vi "FTW-Example-EventLogger.vi"() -> ()   [LabVIEW 2015]
uses:
  source/actor/EventLogger/FTW-Logger.lvclass
  source/actor/Ether/FTW-Ether.lvclass
panel:
  in  "FTW Ether Configuration":string="{\n  \"ApplicationName\": \"Logger Example\",\n  \"ApplicationVersion\": \"0.1.0-1\",\n  \"LoggerAddress\": \"inproc://*\",\n  \"LoggerName\": \"LoggerExample\",\n  \"LoggerDirectory\": \"[UserDesktop]\\\\Logs\",\n  \"LoggerDiskThrashDelay\": 200\n}"
  in  "Logger Configuration":string="{\n  \"Identity\": \"EventLog\",\n  \"InboxAddress\": \"inproc://*\",\n  \"LoggerAddress\": \"\",\n  \"DebugEnableInboxLogging\": false,\n  \"DebugEnableJobLogging\": false,\n  \"DebugShowPanel\": false,\n  \"ApplicationName\": \"LoggerExample\",\n  \"LoggerName\": \"SecondLogger\",\n  \"LoggerDirectory\": \"[UserDesktop]\\\\Logs\",\n  \"LoggerDiskThrashDelay\": 200\n}"
  out "error out":errorcluster
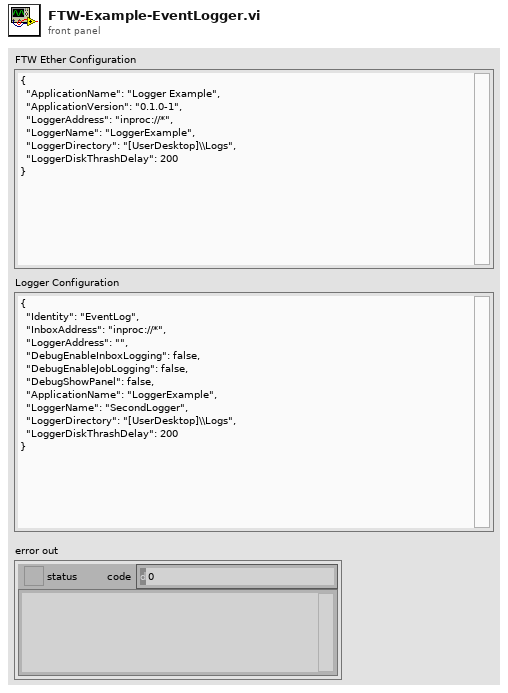
[diagram p1: front panel]
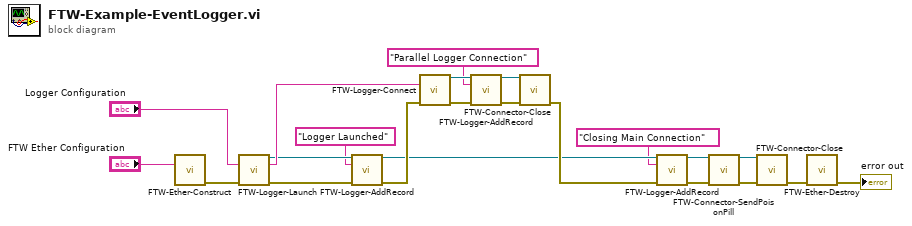
[diagram p0: block diagram]
diagram:
  n1 = call "FTW-Ether-Construct.vi"("FTW Ether Configuration"="FTW Ether Configuration") -> ("error out"=w4:errorcluster)  [unwired: 14 in]
  n2 = call "FTW-Logger-Launch.vi"("FTW Logger Configuration"="Logger Configuration", "error in"=w4) -> ("FTW Logger Connector"=w16:refnum<class "FTW-Logger.lvclass">, "Logger Address"=w18:string, "error out"=w15:errorcluster)  [unwired: 10 in, 1 out]
  n3 = call "FTW-Logger-AddRecord.vi"("FTW Logger Connector"=w16, "Event Type"="Logger Launched", "error in"=w15) -> ("FTW Logger Connector out"=w10:refnum<class "FTW-Logger.lvclass">, "error out"=w14:errorcluster)  [unwired: 10 in, 1 out]
  n4 = call "FTW-Logger-Connect.vi"("Logger Address"=w18, "error in"=w14) -> ("FTW Logger Connector"=w21:refnum<class "FTW-Logger.lvclass">, "error out"=w19:errorcluster)  [unwired: 12 in]
  n5 = call "FTW-Logger-AddRecord.vi"("FTW Logger Connector"=w21, "Event Type"="Parallel Logger Connection", "error in"=w19) -> ("FTW Logger Connector out"=w12:refnum<class "FTW-Logger.lvclass">, "error out"=w11:errorcluster)  [unwired: 10 in, 1 out]
  n6 = call-dynamic "FTW-Connector-Close.vi"("FTW Actor Connector"=w12, "error in"=w11) -> ("error out"=w22:errorcluster)  [unwired: 13 in]
  n7 = call "FTW-Logger-AddRecord.vi"("FTW Logger Connector"=w10, "Event Type"="Closing Main Connection", "error in"=w22) -> ("FTW Logger Connector out"=w8:refnum<class "FTW-Logger.lvclass">, "error out"=w7:errorcluster)  [unwired: 10 in, 1 out]
  n8 = call-dynamic "FTW-Connector-SendPoisonPill.vi"("FTW Actor Connector"=w8, "error in"=w7) -> ("FTW Actor Connector out"=w6:refnum<class "FTW-Logger.lvclass">, "error out"=w5:errorcluster)  [unwired: 8 in, 4 out]
  n9 = call-dynamic "FTW-Connector-Close.vi"("FTW Actor Connector"=w6, "error in"=w5) -> ("error out"=w2:errorcluster)  [unwired: 13 in]
  n10 = call "FTW-Ether-Destroy.vi"("error in"=w2) -> ("error out"=→"error out":errorcluster)  [unwired: 14 in]
